vi "Plugin.Set Thread ID Pool.vi"(10 "Thread ID Pool":refnum<class "ID Pool.lvclass">, 11 "Plugin in":refnum<class "Plugin.lvclass">) -> (3 "Plugin out":refnum<class "Plugin.lvclass">)   [LabVIEW 2017, in "DSF Core.lvlib" / "Plugin.lvclass"]
uses:
  Plugin.lvclass
  Thread Pool/ID Pool.lvclass
  Plugin.lvclass/Plugin.ctl
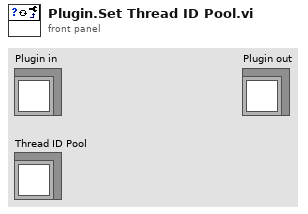
[diagram p1: front panel]
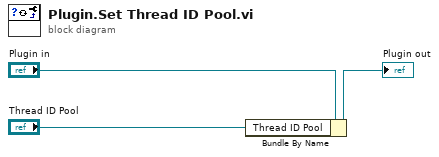
[diagram p0: block diagram]
diagram:
  n1 = Bundle By Name(cluster="Plugin in", "Thread ID Pool"="Thread ID Pool") -> (→"Plugin out":refnum<class "Plugin.lvclass">)
